vi "Image Processing2.vi"() -> ()   [LabVIEW 2016]
uses:
  <vilib>/visionFPGA/Controls/IMAQ FPGA Image Size.ctl
  <vilib>/rvi/Emulation/niFpgaGetClockAttributes.vi
  <vilib>/rvi/Emulation/niFpgaSctlEmulationGetInTimedLoop.vi
  <vilib>/rvi/Emulation/niFpgaEmulationReportErrorSimple.vi
  <vilib>/rvi/Emulation/niFpgaProcessEmulError.vi
  <vilib>/rvi/eio/common/nirviEmuTemplateMethod_errors.vi
  <vilib>/rvi/interface/RandomDataEmulation/niFpgaRandomDataHandleErrors.vi
  <vilib>/rvi/DataTransferAndStorage/Container/Common/niFpgaContainerGetUniqueNameForEmu.vi
  <vilib>/rvi/DataTransferAndStorage/Container/Common/niFpgaContainerSetEmuInfo.vi
  <vilib>/rvi/eio/common/nirviEmuReportErrorAndStop.vi
  <vilib>/rvi/Emulation/niFpgaCriticalErrorInLSC.vi
  <vilib>/eio/EIONode/EIONode.xnode
  <vilib>/rvi/DataTransferAndStorage/Container/XNode/niFpgaContainer.xnode
  <vilib>/rvi/interface/RandomDataEmulation/nirviRandomDataFpgaReadWriteTemplate.vi
  <vilib>/rvi/LocalResourceManager/LocalResourceManager.xnode
panel:
  out "deHeight":u16=240
  out "deWidth":u16=320
  out "Count":u32
  out "OutputType":u8
  out "CanSendImage":bool=TRUE
  out "Mode LED Status":bool=TRUE
  out "Radio LED Status":bool=TRUE
  out "outputExtreme2":bool=TRUE
  out "outputExtreme1":bool=TRUE
  out "outputDOG2":bool=TRUE
  out "outputDOG1":bool=TRUE
  out "Ready For Output":bool=TRUE
  out "StartOfImage":bool=TRUE
  in  "Image Size":T1={"Width"=640, "Height"=480}
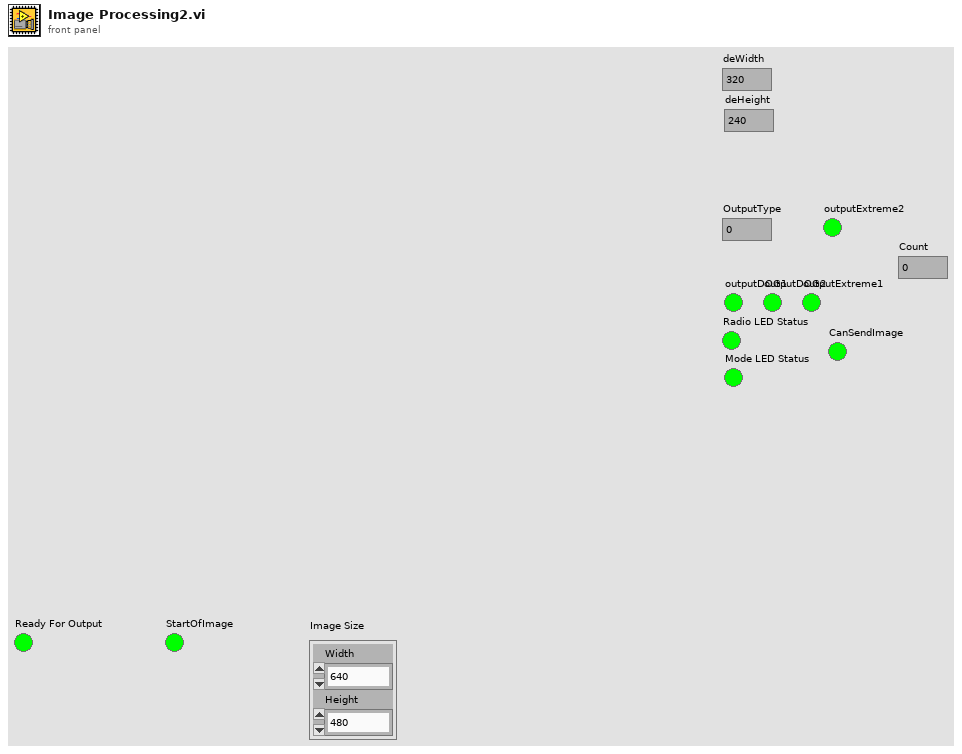
[diagram p1: front panel]
types:
  T1 = typedef "IMAQ FPGA Image Size.ctl" = cluster{"Width":u32, "Height":u32}
  T2 = cluster{"curCol":u16, "curRow":u16, "Width":u32, "Height":u32, "Data Out":u8, bool}
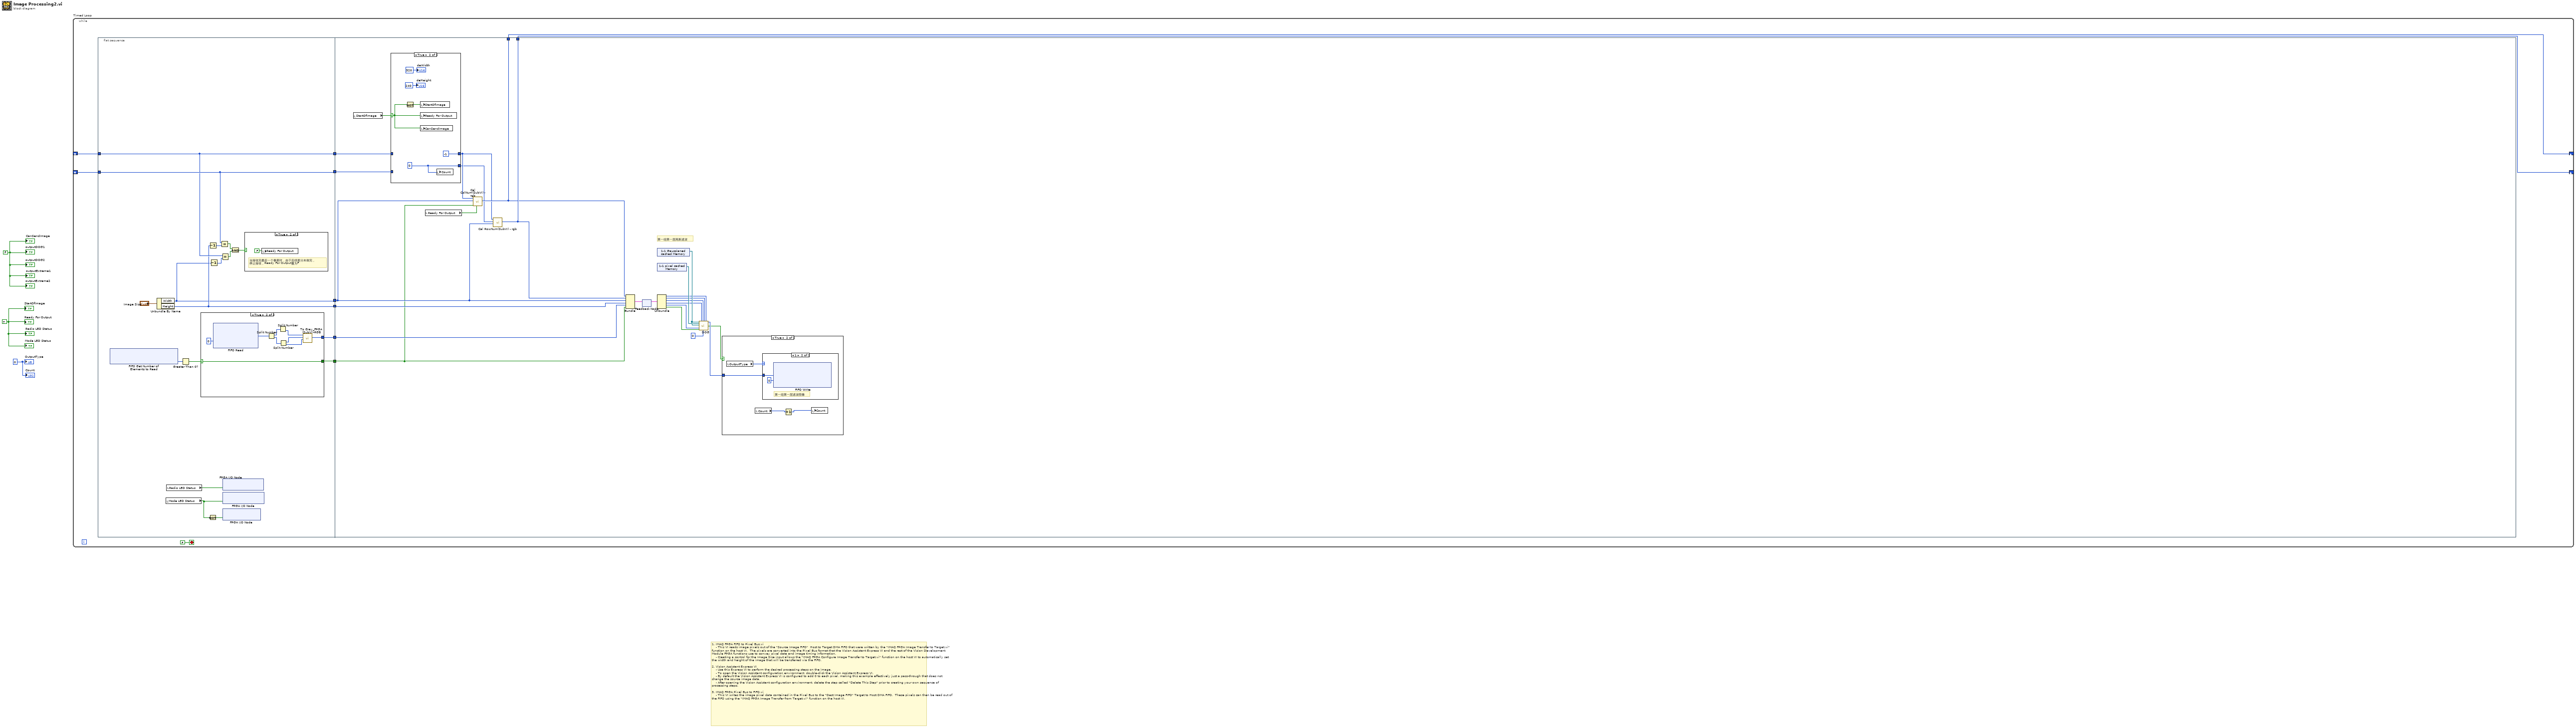
[diagram p0: block diagram]
diagram:
  w1 = FALSE
  w2 = i16 0
  w3 = TRUE ("Ready For Output")
  # "1. IMAQ FPGA FIFO to Pixel Bus.vi\n    - This VI reads image pixels out of the \"Source Image FIFO\"  Host to Target DMA FIFO that were written by the \"IMAQ FPGA Image Transfer to Target.vi\" function on the host VI.  The pixels are converted into the Pixel Bus format that the Vision Assistant Express VI and the rest of the Vision Development Module FPGA functions use to convey pixel data and image timing information.\n    - Creating a control for the Image Size input allows the \"IMAQ FPGA Configure Image Transfer to Target.vi\" function on the host VI to automatically set the width and height of the image that will be transferred via the FIFO.\n\n2. Vision Assistant Express VI\n    - Use this Express VI to perform the desired processing steps on the image.\n    - To open the Vision Assistant configuration environment, double-click the Vision Assistant Express VI.\n    - By default the Vision Assistant Express VI is configured to add 0 to each pixel, making this example effectively just a pass-through that does not change the source image data.\n    - After opening the Vision Assistant configuration environment, delete the step called \"Delete This Step\" prior to creating your own sequence of processing steps.\n\n3. IMAQ FPGA Pixel Bus to FIFO.vi\n    - This VI writes the image pixel data contained in the Pixel Bus to the \"Dest Image FIFO\" Target to Host DMA FIFO.  These pixels can then be read out of the FIFO using the \"IMAQ FPGA Image Transfer from Target.vi\" function on the host VI."
  n1 = while "Timed Loop" {
    shift-right: [w4] -> _
    shift-left: _ -> [w6]
    shift-right: [w5] -> _
    shift-left: _ -> [w8]
    stop <- FALSE stop-if-true
    n2 = flat-sequence {
      tunnel: [w15] -> w13
      tunnel: [w16] -> w12
      tunnel: [w25] -> w11
      tunnel: [w24] -> w10
      tunnel: [w17] -> w9
      tunnel: w8 -> [w17]
      tunnel: [w18] -> w7
      tunnel: w6 -> [w18]
      tunnel: w13 -> [w62]
      tunnel: w12 -> [w61]
      tunnel: w11 -> [w58]
      tunnel: w10 -> [w57]
      tunnel: w9 -> [w44]
      tunnel: w7 -> [w43]
      tunnel: [w50] -> w4
      tunnel: [w49] -> w5
      frame #0 {
        n3 = xnode ("FIFO Get Number of Elements to Read")() -> ("Number of Elements to Read"=w27:u32)  [unwired: 1 in, 1 out]
        n4 = Unbundle By Name("Image Size") -> ("Width"=w15:u32, "Height"=w16:u32)
        n5 = local read "Mode LED Status"() -> (w30:bool)
        n6 = local read "Radio LED Status"() -> (w28:bool)
        n7 = Greater Than 0?(x=w27) -> (x > 0?=w26:bool)
        n8 = case shown="True" w26 {
          selector: w26 -> [w33 w34]
          tunnel: [_ w35] -> w25
          tunnel: [w33 w34] -> w24
          frame False {
          }
          frame True {
            n9 = xnode ("FIFO Read")("Timeout"=0) -> ("Element"=w42:u32)  [unwired: 1 in, 2 out]
            n10 = Split Number(x=w42) -> (hi(x)=w40:u16, lo(x)=w41:u16)
            n11 = Split Number(x=w40) -> (lo(x)=w39:u8)  [unwired: 1 out]
            n12 = Split Number(x=w41) -> (hi(x)=w38:u8, lo(x)=w37:u8)
            n13 = call "To Gray_FPGA (SubVI)-RGB.vi"("B"=w37, "G"=w38, "R"=w39) -> ("Data Out"=w35:u8)  [unwired: 8 in]
          }
        }
        n14 = Not(x=w30) -> (.not. x?=w29:bool)
        n15 = Decrement(x=w16) -> (x-1=w21:u32)
        n16 = Decrement(x=w15) -> (x-1=w22:u32)
        n17 = Equal?(x=w18, y=w21) -> (x = y?=w19:bool)
        n18 = Equal?(x=w17, y=w22) -> (x = y?=w20:bool)
        n19 = xnode "FPGA I/O Node"("Radio LED Green"=w28) -> ()  [unwired: 1 in, 1 out]
        n20 = xnode "FPGA I/O Node"("Mode LED Green"=w30) -> ()  [unwired: 1 in, 1 out]
        n21 = xnode "FPGA I/O Node"("Mode LED Red"=w29) -> ()  [unwired: 1 in, 1 out]
        n22 = And(x=w19, y=w20) -> (x .and. y?=w23:bool)
        n23 = case shown="True" w23 {
          frame False {
          }
          frame True {
            # "当接收完最后一个像素时，由于后续差分未做完，\n停止接收，Ready For Output置为F"
            n24 = local write "Ready For Output"(FALSE ("Ready For Output")) -> ()
          }
        }
      }
      frame #1 {
        # "第一组第一层高斯滤波"
        n25 = local read "StartOfImage"() -> (w45:bool)
        n26 = case shown="True" w45 {
          selector: w45 -> [_ w73]
          tunnel: w44 -> [w69 _]
          tunnel: w43 -> [w68 _]
          tunnel: [w69 i16 -1] -> w47
          tunnel: [w68 w72] -> w46
          frame False {
          }
          frame True {
            w72 = i16 0
            n27 = Not(x=w73) -> (.not. x?=w74:bool)
            n28 = local write "StartOfImage"(w74) -> ()
            n29 = local write "Ready For Output"(w73) -> ()
            n30 = local write "CanSendImage"(w73) -> ()
            n31 = local write "Count"(w72) -> ()
            "deWidth" <- i16 320
            "deHeight" <- i16 240
          }
        }
        n32 = local read "Ready For Output"() -> (w48:bool)
        n33 = call "Cal ColNum(SubVI) - rgb.vi"("Ready For Input"=w48, "DV"=w57, "Width"=w62, "preCol"=w47) -> ("curCol"=w49:u16)  [unwired: 7 in]
        n34 = call "Cal RowNum(SubVI) - rgb.vi"("Width"=w62, "preRow"=w46, "preCol"=w47) -> ("curRow"=w50:u16)  [unwired: 8 in]
        n35 = Bundle("curCol"=w49, "curRow"=w50, "Width"=w62, "Height"=w61, "Data Out"=w58, w57) -> (w64:T2)  [unwired: 1 in]
        n36 = feedback #1() -> (w63:T2)  [unwired: 1 in]
        n37 = feedback-in #1(w64) -> ()
        n38 = xnode "1-1 Gaussianed cached Memory"() -> ("Memory Out"=w67:refnum<k21>)
        n39 = xnode "1-1 pixel cached Memory"() -> ("Memory Out"=w66:refnum<k21>)
        n40 = Unbundle(w63) -> ("curCol"=w56:u16, "curRow"=w55:u16, "Width"=w54:u32, "Height"=w53:u32, "Data Out"=w60:u8, w59:bool)
        n41 = call "DOG.vi"("Gaussianed cached Memory"=w67, "pixel cached Memory"=w66, "preGaussianed cached Memory"=w67, "Data in"=w60, "DV in"=w59, "Height"=w53, "Width"=w54, "DelayRowCount"=i16 0, "Rows"=w55, "Cols"=w56) -> ("GaussianFilterData out"=w52:u8, "DV out"=w51:bool)  [unwired: 6 in, 2 out]
        n42 = case shown="True" w51 {
          tunnel: w52 -> [_ w79]
          frame False {
          }
          frame True {
            n43 = local read "OutputType"() -> (w78:u8)
            n44 = local read "Count"() -> (w77:u32)
            n45 = case shown="1" w78 {
              tunnel: w79 -> [_ w80]
              frame 0, Default {
              }
              frame 1 {
                # "第一组第一层滤波图像"
                n46 = xnode ("FIFO Write")("Element"=w80, "Timeout"=0) -> ()  [unwired: 1 in, 2 out]
              }
            }
            n47 = Increment(x=w77) -> (x+1=w76:u32)
            n48 = local write "Count"(w76) -> ()
          }
        }
      }
    }
  }
  "StartOfImage" <- w3
  "Ready For Output" <- w3
  "outputDOG1" <- w1
  "outputDOG2" <- w1
  "outputExtreme1" <- w1
  "outputExtreme2" <- w1
  "Radio LED Status" <- w3
  "Mode LED Status" <- w3
  "CanSendImage" <- w1
  "OutputType" <- w2
  "Count" <- w2
